vi "Get or Set DAQmx CFG Message Data.vi"(6 "mode":enum16{"Get", "Set"}(ring), 7 "DAQmx Cfg in":T1 {"Run Mode" items=["Run Once", "Continuously"]; "Block Size" min=0; "Sample Rate (Hz)" min=0.0; "Trigger Type" items=["None", "Analog Reference"]; "Channel Table"."input terminal configuration" items=["default"=-1, "RSE"=10083, "NRSE"=10078, "Differential"=10106, "Pseudodifferential"=12529]; "Channel Table"."Channel Type" items=["Voltage (V)"=0, "Charge (C)"=9, "-"=99, "SPL (Pa)"=3, "Force (lbf)"=6, "Force (N)"=1, "Acceleration (g) - IEPE"=2, "Acceleration (g) - Charge"=12, "Acceleration (g) - 4 wire DC Voltage"=22, "Velocity (in/s)"=7, "Velocity (mm/s)"=8, "Prox Probe (mil)"=4, "Prox Probe (mm)"=5]}, 8 "error in (no error)":errorcluster, 9 "log duration":dbl, 10 "log directory":path, 11 "message data in":variant) -> (0 "error out":errorcluster, 1 "log duration out":dbl, 2 "log directory out":path, 3 "message data out":variant, 5 "DAQmx Cfg out":T1 {"Run Mode" items=["Run Once", "Continuously"]; "Block Size" min=0; "Sample Rate (Hz)" min=0.0; "Trigger Type" items=["None", "Analog Reference"]; "Channel Table"."input terminal configuration" items=["default"=-1, "RSE"=10083, "NRSE"=10078, "Differential"=10106, "Pseudodifferential"=12529]; "Channel Table"."Channel Type" items=["Voltage (V)"=0, "Charge (C)"=9, "-"=99, "SPL (Pa)"=3, "Force (lbf)"=6, "Force (N)"=1, "Acceleration (g) - IEPE"=2, "Acceleration (g) - Charge"=12, "Acceleration (g) - 4 wire DC Voltage"=22, "Velocity (in/s)"=7, "Velocity (mm/s)"=8, "Prox Probe (mil)"=4, "Prox Probe (mm)"=5]})   [LabVIEW 2024]
uses:
  DSA_CFG_ACQ.lvlib
  Dynamic Signal Acquisition (Interactive) UI/SFPDAQmx Channel Info.ctl
  Dynamic Signal Acquisition (Interactive) UI/Dynamic Signal Acquisition (Interactive) UI.lvlib
  <vilib>/addons/Sound and Vibration/svt_DAQmx/Configuration XControl/Controls/svx_DAQ_Trigger_Slope.ctl
  <vilib>/addons/Sound and Vibration/svt_DAQmx/Configuration XControl/SVX NI-DAQmx AI Configuration XControl.xctl
  Dynamic Signal Acquisition (Interactive) UI/SFPDAQ Configuration.ctl
  <vilib>/addons/Sound and Vibration/svt_DAQmx/subVIs/Run Mode.ctl
  <vilib>/addons/Sound and Vibration/svt_DAQmx/subVIs/SV_DAQmx.lvlib
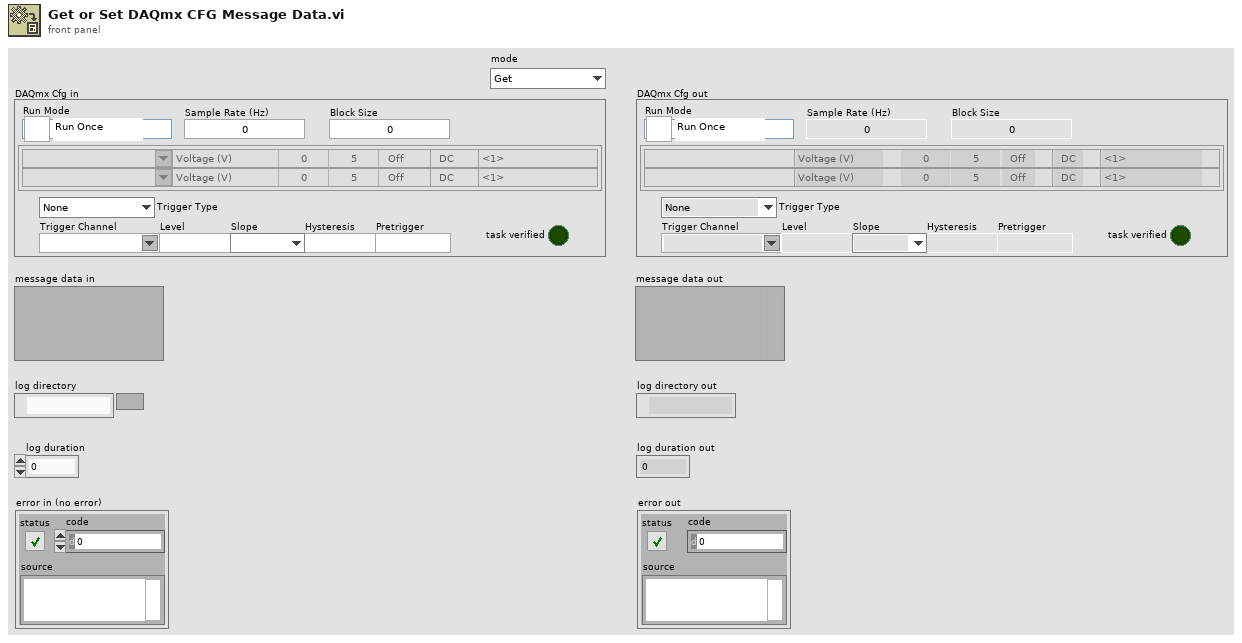
[diagram p1: front panel]
types:
  T1 = typedef "Dynamic Signal Acquisition (Interactive) UI.lvlib/SFPDAQ Configuration.ctl" = cluster{"Sample Rate (Hz)":dbl, "Block Size":i32, "Channel Table":T2[], "Trigger Type":u16, "Trigger Channel":string, "Level":dbl, "Pretrigger":i32, "Hysteresis":dbl, "Slope":T3, "Run Mode":T4, "task verified":bool}
  T2 = typedef "Dynamic Signal Acquisition (Interactive) UI.lvlib/SFPDAQmx Channel Info.ctl" = cluster{"DAQmx Channel":tag, "Channel Type":u16, "Max":dbl, "Sensitivity":dbl, "Coupling":enum16{"AC", "DC"}, "input terminal configuration":i32, "excitation":enum16{"Off", "Min", "Max"}}
  T3 = typedef "SVX NI-DAQmx AI Configuration XControl.xctl/svx_DAQ_Trigger_Slope.ctl" = enum16{"Falling", "Rising"}
  T4 = typedef "SV_DAQmx.lvlib/Run Mode.ctl" = u16
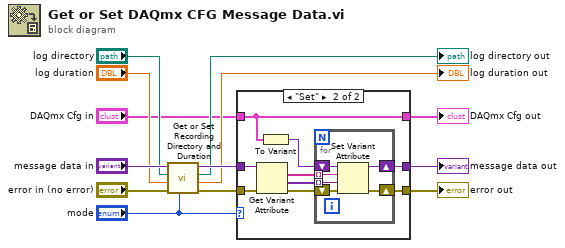
[diagram p0: block diagram]
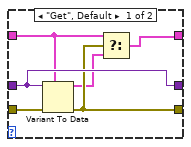
[diagram p2: hidden frame]
diagram:
  n1 = call "Get or Set Recording Directory and Duration.vi"("mode"="mode", "error in (no error)"="error in (no error)", "log duration in"="log duration", "log directory in"="log directory", "Message Data"="message data in") -> ("error out"=w3:errorcluster, "log duration out"=→"log duration out":dbl, "log directory out"=→"log directory out":path, "Variant"=w13:variant)  [unwired: 1 in]
  n2 = case shown="\"Set\"" "mode" {
    tunnel: w13 -> [w18 w28]
    tunnel: [w17 w21] -> w7
    tunnel: [w14 w26] -> w5
    tunnel: "DAQmx Cfg in" -> [w16 w26]
    tunnel: w3 -> [w19 w27]
    tunnel: [w18 w20] -> w1
    frame "Get", Default {
      n3 = Variant To Data(error in=w19, type=w16, Variant=w18) -> (data=w15:T1, error out=w17:errorcluster)
      n4 = Select(t=w16, s=w17, f=w15) -> (s? t:f=w14:T1)
    }
    frame "Set" {
      n5 = Get Variant Attribute(Variant=w28, error in=w27) -> (names=w24:string[], values=w23:variant[], error out=w22:errorcluster)  [unwired: 2 in, 1 out]
      n6 = To Variant(anything=w26) -> (Variant=w25:variant)
      n7 = for {
        shift-right: [w33] -> w20
        shift-left: w25 -> [w34]
        tunnel: w24 -> [w32] mode=indexing
        tunnel: w23 -> [w31] mode=indexing
        shift-right: [w29] -> w21
        shift-left: w22 -> [w30]
        n8 = Set Variant Attribute(Variant=w34, name=w32, value=w31, error in=w30) -> (Variant out=w33:variant, error out=w29:errorcluster)  [unwired: 1 out]
      }
    }
  }
  "error out" <- w7
  "DAQmx Cfg out" <- w5
  "message data out" <- w1
